vi "Teleop.vi"(10 "Match Info":T1={"Autonomous Elapsed Seconds"=0.0, "TeleOp Elapsed Seconds"=0.0, "Disabled Elapsed Seconds"=0.0, "Visited Autonomous"=FALSE, "Visited TeleOp"=FALSE, "Visited Disabled"=FALSE, "Autonomous Settings"={"Autonomous Style"=enum."Independent", "VI Refnum"=refnum}}, 11 "Call Context":T2) -> ()   [LabVIEW 2015]
doc: "This VI is called for each TeleOp packet received from the DS where the robot is not disabled. It is often used to read from the joysticks and update I/O or to update setpoints for timed control loops. It should complete and return within 20 milliseconds or it may miss DS packets."
uses:
  <vilib>/Rock Robotics/WPI/DriverStation/WPI_DriverStationDerivedRobotMode.ctl
  <vilib>/Rock Robotics/WPI/DriverStation/WPI_DriverStationMatch Info.ctl
  <vilib>/Rock Robotics/WPI/Utilities/WPI_GetSetVariantRefNum.vi
  <vilib>/Rock Robotics/Network Tables/SD Write Number.vi
  Robot Global Data.vi
  <vilib>/Rock Robotics/WPI/Solenoid/Deprecated/WPI_SolenoidSetBool.vi
  <vilib>/addons/control/pid/NI_PID_pid.lvlib
  <vilib>/addons/control/pid/pid.llb/PID (DBL).vi
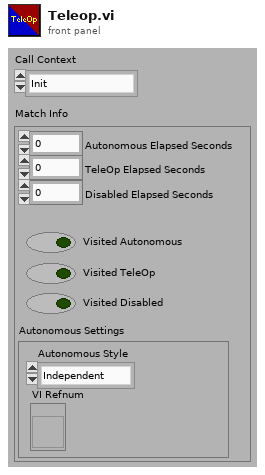
[diagram p1: front panel]
types:
  T1 = typedef "WPI_DriverStationMatch Info.ctl" = cluster{"Autonomous Elapsed Seconds":dbl, "TeleOp Elapsed Seconds":dbl, "Disabled Elapsed Seconds":dbl, "Visited Autonomous":bool, "Visited TeleOp":bool, "Visited Disabled":bool, "Autonomous Settings":cluster{"Autonomous Style":enum16{"Iterative", "Independent"}, "VI Refnum":refnum<vi>}}
  T2 = typedef "WPI_DriverStationDerivedRobotMode.ctl" = enum16{"Init", "Execute", "Stop"}
  T3 = typedef "WPI_SolenoidDevRef.ctl" = cluster{"DevStatus":errorcluster, "Pneumatics Control Module":u8, "Forward Solenoid Channel":T4, "Reverse Solenoid Channel":T4}
  T4 = typedef "WPI_SolenoidChannel.ctl" = enum8{"Solenoid 0", "Solenoid 1", "Solenoid 2", "Solenoid 3", "Solenoid 4", "Solenoid 5", "Solenoid 6", "Solenoid 7", "Invalid"}
  T5 = typedef "WPI_RobotDriveDevRef.ctl" = cluster{"DevStatus":errorcluster, "Motors[]":T6[], "Square Inputs":bool, "Max Output":dbl}
  T6 = typedef "WPI_MotorControlDeviceRef.ctl" = cluster{"DeviceStatus":errorcluster, "Type":T7, "PWM":cluster{"PWM Channel":T8, "DeadBand":T9}, "CAN":cluster{"Device Number":u8, "Control Mode":T10, "Semaphore":T11, "Max Vout":dbl, "TalonSRX Control Mode":T12}, "Invert":bool}
  T7 = typedef "WPI_MotorControlType.ctl" = enum16{"PWM", "CAN", "CANTalonSRX"}
  T8 = typedef "FPGA_DIOPWMChannel.ctl" = enum8{"PWM 0", "PWM 1", "PWM 2", "PWM 3", "PWM 4", "PWM 5", "PWM 6", "PWM 7", "PWM 8", "PWM 9", "PWM MXP 0", "PWM MXP 1", "PWM MXP 2", "PWM MXP 3", "PWM MXP 4", "PWM MXP 5", "PWM MXP 6", "PWM MXP 7", "PWM MXP 8", "PWM MXP 9", "Invalid"}
  T9 = typedef "WPI_PWMDeadband.ctl" = cluster{"Name":string, "maxPositivePwm":i32, "minPositivePwm":i32, "centerPwm":i32, "maxNegativePwm":i32, "minNegativePwm":i32, "angularRange":u16}
  T10 = typedef "WPI_CANJaguar_ControlMode.ctl" = enum8{"Percent VBus", "Current", "Speed", "Position", "Voltage"}
  T11 = typedef "Semaphore RefNum" = refnum<k1>
  T12 = typedef "WPI_CANTalonSRX_APIControlMode.ctl" = enum8{"Percent VBus", "Speed", "Position", "Slave", "Unchanged / Invalid", "Voltage Compensation", "Current", "Motion Profile"}
  T13 = typedef "WPI_CANTalonSRX_GlobalStatus.ctl" = cluster{"Applied Throttle":dbl, "Module Enabled":bool, "CAN Error":errorcluster, "Closed Loop Error":dbl, "Forward Limit Switch Closed":bool, "Reverse Limit Switch Closed":bool, "Sensor Position":dbl, "Sensor Velocity":dbl, "Current":dbl, "Sticky Fault - Over Temp":bool, "Sticky Fault - Under Voltage":bool, "Sticky Fault - Forward Limit":bool, "Sticky Fault - Reverse Limit":bool, "Sticky Fault - Forward Soft Limit":bool, "Sticky Fault - Reverse Soft Limit":bool, "Brake is Enabled":bool, "Encoder Position":dbl, "Encoder Velocity":dbl, "Encoder Index Count":dbl, "Encoder A Pin State":bool, "Encoder B Pin State":bool, "Encoder Index Pin State":bool, "Analog In":dbl, "Analog In Velocity":dbl, "Temperature (C)":dbl, "Battery Voltage":dbl, "Control 5 Is Supported":bool, "Current Profile Slot Select":dbl, "Pos Div 8":bool, "Vel Div 4":bool, "Pulse Width Position":i32, "Pulse Width Velocity":i32, "Pulse Width Rise To Rise (us)":i32, "Pulse Width Rise To Fall (us)":i32, "Mot Prof Active Is Under Run":bool, "Mot Prof Active Has Under Run":bool, "Mot Prof Active Is Last":bool, "Mot Prof Active Velocity Only":bool, "Mot Prof Active Is Valid":bool, "Mot Prof Buffer Is Full":bool, "Mot Prof Active Profile Slot Select":i32, "Mot Prof NextID":i32, "Mot Prof Count":i32, "Mot Prof Active Velocity":dbl, "Mot Prof Active Position":dbl, "Mot Prof Output Enable":i32}
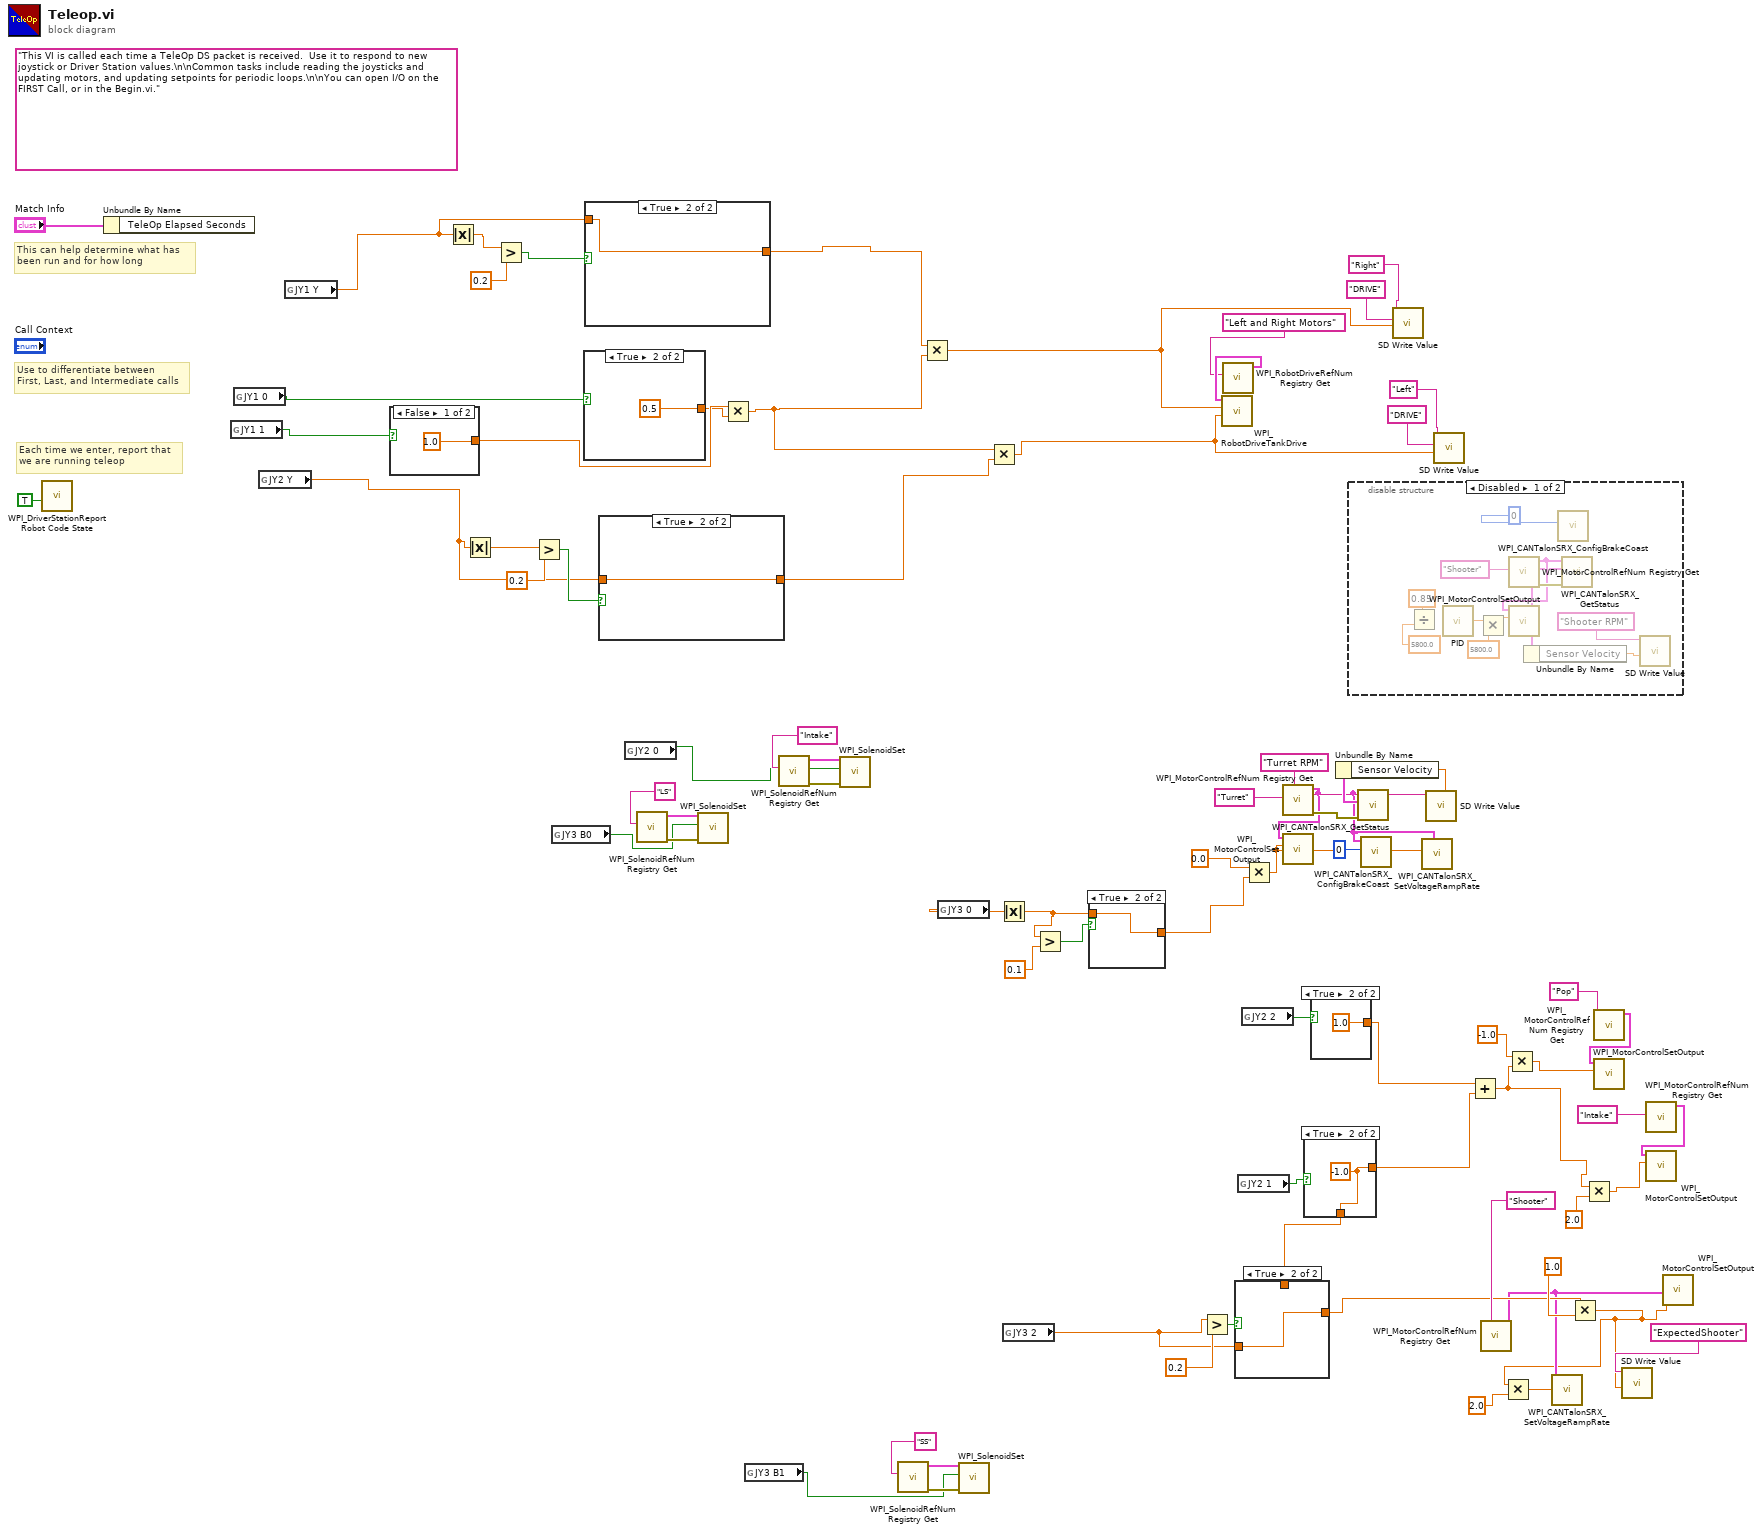
[diagram p0: block diagram]
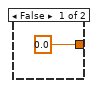
[diagram p2: hidden frame]
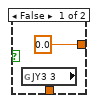
[diagram p4: hidden frame]
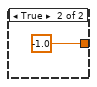
[diagram p5: hidden frame]
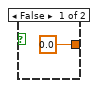
[diagram p7: hidden frame]
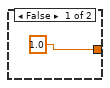
[diagram p8: hidden frame]
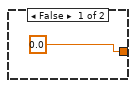
[diagram p9: hidden frame]
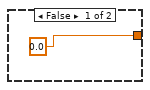
[diagram p10: hidden frame]
diagram:
  (unwired) "This VI is called each time a TeleOp DS packet is received.  Use it to respond to new joystick or Driver Station values.\n\nCommon tasks include reading the joysticks and updating motors, and updating setpoints for periodic loops.\n\nYou can open I/O on the FIRST Call, or in the Begin.vi."
  # "Each time we enter, report that\nwe are running teleop"
  # "Use to differentiate between\nFirst, Last, and Intermediate calls"
  # "This can help determine what has\nbeen run and for how long"
  n1 = call <vilib>:"WPI_DriverStationReport Robot Code State.vi"("TeleOp"=TRUE ("Autonomous")) -> ()  [unwired: 10 in, 1 out]
  n2 = Unbundle By Name("Match Info") -> ()  [unwired: 1 out]
  n3 = global read "Robot Global Data.vi" "JY1 1"() -> (w40:bool)
  n4 = global read "Robot Global Data.vi" "JY1 0"() -> (w66:bool)
  n5 = global read "Robot Global Data.vi" "JY2 Y"() -> (w67:dbl)
  n6 = global read "Robot Global Data.vi" "JY1 Y"() -> (w68:dbl)
  n7 = case shown="False" w40 {
    tunnel: [1.0 -1.0] -> w39
    frame False {
    }
    frame True {
    }
  }
  n8 = Absolute Value(x=w68) -> (abs(x)=w70:dbl)
  n9 = Absolute Value(x=w67) -> (abs(x)=w69:dbl)
  n10 = Greater?(x=w70, y=0.2) -> (0:w74:bool)
  n11 = Greater?(x=w69, y=0.2) -> (0:w72:bool)
  n12 = global read "Robot Global Data.vi" "JY3 B0"() -> (w43:bool)
  n13 = case shown="True" w66 {
    tunnel: [1.0 0.5] -> w37
    frame False {
    }
    frame True {
    }
  }
  n14 = case shown="True" w74 {
    tunnel: [0.0 w82] -> w60
    tunnel: w68 -> [_ w82]
    frame False {
    }
    frame True {
    }
  }
  n15 = case shown="True" w72 {
    tunnel: [0.0 w84] -> w61
    tunnel: w67 -> [_ _]
    tunnel: w67 -> [_ w84]
    frame False {
    }
    frame True {
    }
  }
  n16 = global read "Robot Global Data.vi" "JY2 0"() -> (w44:bool)
  n17 = call <vilib>:"WPI_SolenoidRefNum Registry Get.vi"("refnum name"="LS") -> ("error out"=w53:errorcluster, "SolenoidDevRef"=w54:T3)  [unwired: 9 in]
  n18 = call-poly <vilib>:"WPI_SolenoidSet.vi"("error in (no error)"=w53, "Value"=w43, "SolenoidDevRef"=w54) -> ()  [unwired: 9 out]
  n19 = Multiply(x=w39, y=w37) -> (x*y=w38:dbl)
  n20 = global read "Robot Global Data.vi" "JY3 B1"() -> (w7:bool)
  n21 = call <vilib>:"WPI_SolenoidRefNum Registry Get.vi"("refnum name"="Intake") -> ("error out"=w50:errorcluster, "SolenoidDevRef"=w51:T3)  [unwired: 9 in]
  n22 = call-poly <vilib>:"WPI_SolenoidSet.vi"("error in (no error)"=w50, "Value"=w44, "SolenoidDevRef"=w51) -> ()  [unwired: 9 out]
  n23 = call <vilib>:"WPI_SolenoidRefNum Registry Get.vi"("refnum name"="SS") -> ("error out"=w9:errorcluster, "SolenoidDevRef"=w10:T3)  [unwired: 9 in]
  n24 = Multiply(x=w60, y=w38) -> (x*y=w48:dbl)
  n25 = global read "Robot Global Data.vi" "JY3 0"() -> (w2:dbl)
  n26 = call-poly <vilib>:"WPI_SolenoidSet.vi"("error in (no error)"=w9, "Value"=w7, "SolenoidDevRef"=w10) -> ()  [unwired: 9 out]
  n27 = Multiply(x=w38, y=w61) -> (x*y=w47:dbl)
  n28 = Absolute Value(x=w2) -> (abs(x)=w1:dbl)
  n29 = global read "Robot Global Data.vi" "JY3 2"() -> (w21:dbl)
  n30 = Greater?(x=w1, y=0.1) -> (0:w5:bool)
  n31 = case shown="True" w5 {
    tunnel: [0.0 w86] -> w4
    tunnel: w1 -> [_ w86]
    frame False {
    }
    frame True {
    }
  }
  n32 = Greater?(x=w21, y=0.2) -> (0:w11:bool)
  n33 = call <vilib>:"WPI_RobotDriveRefNum Registry Get.vi"("refnum name"="Left and Right Motors") -> ("RobotDriveDevRef"=w58:T5)  [unwired: 9 in, 1 out]
  n34 = call <vilib>:"WPI_RobotDriveTankDrive.vi"("Right axis value"=w47, "Left axis value"=w48, "RobotDriveDevRef"=w58) -> ()  [unwired: 6 in, 3 out]
  n35 = global read "Robot Global Data.vi" "JY2 1"() -> (w33:bool)
  n36 = global read "Robot Global Data.vi" "JY2 2"() -> (w34:bool)
  n37 = Multiply(x=0.0, y=w4) -> (x*y=w20:dbl)
  n38 = call <vilib>:"WPI_MotorControlRefNum Registry Get.vi"("refnum name"="Turret") -> ("error out"=w42:errorcluster, "MotorControlDevRef"=w19:T6)  [unwired: 9 in]
  n39 = call <vilib>:"WPI_MotorControlSetOutput.vi"("Output"=w20, "MotorControlDevRef"=w19) -> ()  [unwired: 7 in, 3 out]
  n40 = case shown="True" w33 {
    tunnel: [0.0 w89] -> w31
    tunnel: [w87 w89] -> w22
    frame False {
      n41 = global read "Robot Global Data.vi" "JY3 3"() -> (w87:dbl)
    }
    frame True {
      w89 = -1.0
    }
  }
  n42 = case shown="True" w11 {
    tunnel: [w90 w91] -> w23
    tunnel: w22 -> [w90 _]
    tunnel: w21 -> [_ w91]
    frame False {
    }
    frame True {
    }
  }
  n43 = case shown="True" w34 {
    tunnel: [0.0 1.0] -> w32
    frame False {
    }
    frame True {
    }
  }
  n44 = disable-structure shown="Disabled" {
    frame Disabled {
      n45 = Divide(x=0.85, y=5800.0) -> ()  [unwired: 1 out]
      n46 = call-poly <vilib>:"PID.vi"() -> ("output"=w97:dbl)  [unwired: 10 in, 1 out]
      n47 = Multiply(x=w97, y=5800.0) -> (x*y=w104:dbl)
      n48 = call <vilib>:"WPI_MotorControlRefNum Registry Get.vi"("refnum name"="Shooter") -> ("error out"=w102:errorcluster, "MotorControlDevRef"=w100:T6)  [unwired: 9 in]
      n49 = call <vilib>:"WPI_MotorControlSetOutput.vi"("Output"=w104, "MotorControlDevRef"=w100) -> ()  [unwired: 7 in, 3 out]
      n50 = call <vilib>:"WPI_CANTalonSRX_ConfigBrakeCoast.vi"("Brake / Coast Mode"=0) -> ()  [unwired: 9 in, 2 out]
      n51 = call <vilib>:"WPI_CANTalonSRX_GetStatus.vi"("error in (no error)"=w102, "CAN Talon SRX Ref"=w100) -> ("Talon SRX Status"=w99:T13)  [unwired: 7 in, 2 out]
      n52 = Unbundle By Name(w99) -> ("Sensor Velocity"=w95:dbl)
      n53 = call-poly <vilib>:"SD Write Value.vi"("Numeric"=w95, "Name"="Shooter RPM") -> ()  [unwired: 8 in, 2 out]
    }
    frame Enabled {
    }
  }
  n54 = call <vilib>:"WPI_CANTalonSRX_GetStatus.vi"("error in (no error)"=w42, "CAN Talon SRX Ref"=w19) -> ("Talon SRX Status"=w56:T13)  [unwired: 7 in, 2 out]
  n55 = Unbundle By Name(w56) -> ("Sensor Velocity"=w30:dbl)
  n56 = call <vilib>:"WPI_CANTalonSRX_ConfigBrakeCoast.vi"("Brake / Coast Mode"=0, "CAN Talon SRX Ref"=w19) -> ()  [unwired: 8 in, 2 out]
  n57 = call-poly <vilib>:"SD Write Value.vi"("Numeric"=w48, "Table Prefix"="DRIVE", "Name"="Right") -> ()  [unwired: 7 in, 2 out]
  n58 = call <vilib>:"WPI_CANTalonSRX_SetVoltageRampRate.vi"("Throttle Ramp Rate (percent/s)"=w20, "CAN Talon SRX Ref"=w19) -> ()  [unwired: 8 in, 2 out]
  n59 = call-poly <vilib>:"SD Write Value.vi"("Numeric"=w30, "Name"="Turret RPM") -> ()  [unwired: 8 in, 2 out]
  n60 = call-poly <vilib>:"SD Write Value.vi"("Numeric"=w47, "Table Prefix"="DRIVE", "Name"="Left") -> ()  [unwired: 7 in, 2 out]
  n61 = Add(x=w32, y=w31) -> (x+y=w15:dbl)
  n62 = call <vilib>:"WPI_MotorControlRefNum Registry Get.vi"("refnum name"="Shooter") -> ("MotorControlDevRef"=w18:T6)  [unwired: 9 in, 1 out]
  n63 = Multiply(x=-1.0, y=w15) -> (x*y=w29:dbl)
  n64 = Multiply(x=w23, y=1.0) -> (x*y=w14:dbl)
  n65 = Multiply(x=w14, y=2.0) -> (x*y=w13:dbl)
  n66 = call <vilib>:"WPI_CANTalonSRX_SetVoltageRampRate.vi"("Throttle Ramp Rate (percent/s)"=w13, "CAN Talon SRX Ref"=w18) -> ()  [unwired: 8 in, 2 out]
  n67 = Multiply(x=w15, y=2.0) -> (x*y=w16:dbl)
  n68 = call <vilib>:"WPI_MotorControlRefNum Registry Get.vi"("refnum name"="Pop") -> ("MotorControlDevRef"=w45:T6)  [unwired: 9 in, 1 out]
  n69 = call <vilib>:"WPI_MotorControlSetOutput.vi"("Output"=w29, "MotorControlDevRef"=w45) -> ()  [unwired: 7 in, 3 out]
  n70 = call-poly <vilib>:"SD Write Value.vi"("Numeric"=w14, "Name"="ExpectedShooter") -> ()  [unwired: 8 in, 2 out]
  n71 = call <vilib>:"WPI_MotorControlRefNum Registry Get.vi"("refnum name"="Intake") -> ("MotorControlDevRef"=w35:T6)  [unwired: 9 in, 1 out]
  n72 = call <vilib>:"WPI_MotorControlSetOutput.vi"("Output"=w16, "MotorControlDevRef"=w35) -> ()  [unwired: 7 in, 3 out]
  n73 = call <vilib>:"WPI_MotorControlSetOutput.vi"("Output"=w14, "MotorControlDevRef"=w18) -> ()  [unwired: 7 in, 3 out]
